vi "Compute Calibrated Phasor Array.vi"(6 "Phasor Calibration Data":T7, 7 "Phasor Calculation":T1, 8 "Error In":errorcluster, 9 "Gates Definitions":T4={"First Gate: t1"=0.0, "Gate Width: W"=0.0, "Gate Step: d"=0.0, "# Gates: G"=0.0, "Use Gate Center"=FALSE, "Frames/Image: F"=50, "Gates/Frame: L"=0, "Bits/Frame: q"=0, "Multiplicity: p"=0, "Gate Type"=enum."Square", "Gate Edge s"=4.0, "Gate Top Slope"=4.0, "Reversed Sawtooth?"=FALSE, "Computation"=FALSE, "User-defined Gate"={"X Array"=[], "Y Array"=[]}, "Tolerance"=50.0, "Integration"=enum."Item 0", "# Steps"=50.0, "Type of User-defined Function"=enum."Gate"}, 10 "Decay Definition":T2={"offset: t0"=0.0, "period: T"=0.0, "lifetime: tau"=0.0, "Incident Signal: I"=0.5, "Normalized Decays"=FALSE, "IRF Model"=enum."Dirac", "IRF Parameter 1"=0.0}, 11 "Lifetime Array":ext[](array[numeric])) -> (0 "Error Out":errorcluster, 1 "Calibrated s Array":ext[](array[numeric]), 2 "Calibrated g Array":ext[](array[numeric]), 3 "True Lifetime Array":ext[](array[numeric]), 4 "# Rejected Pairs":i32, 5 "CPU (s)":dbl)   [LabVIEW 2019]
uses:
  Phasor Calibration Data.ctl
  Gate Definitions.ctl
  Gate Type.ctl
  XY Plot Data.ctl
  Decay Definiton.ctl
  IRF Model.ctl
  Phasor Calculation Type.ctl
  SEPXP Globals.vi
panel:
  out "Uncalibrated Phasors":cxt[](array[numeric])
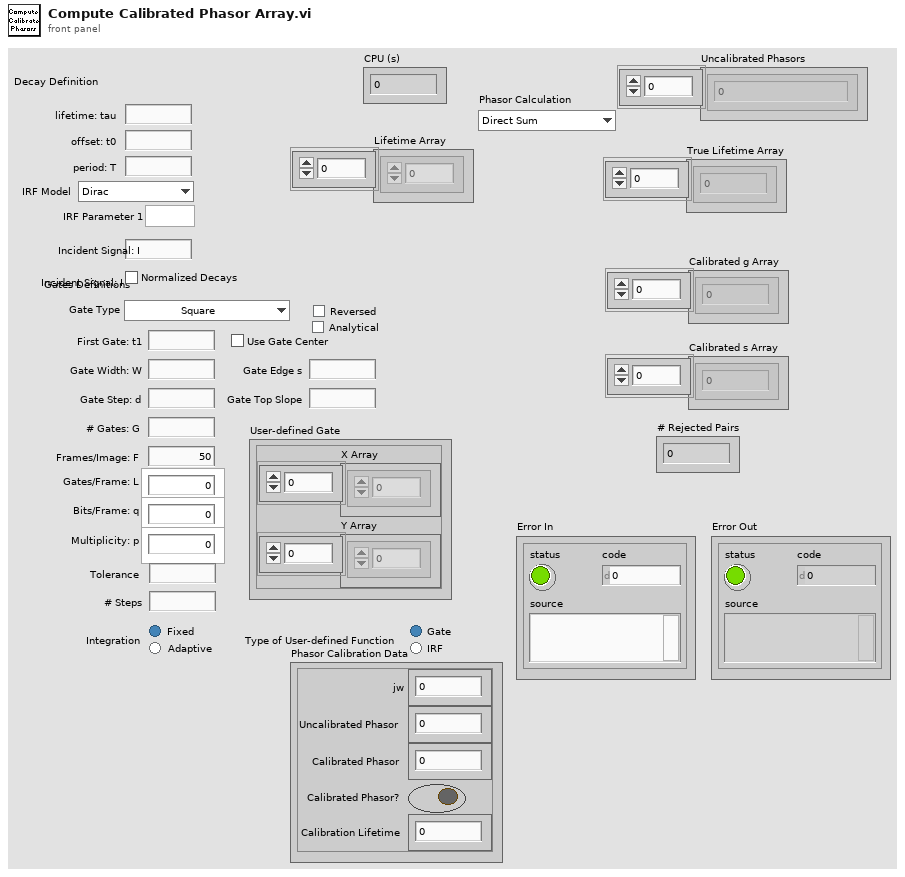
[diagram p1: front panel]
types:
  T1 = typedef "Phasor Calculation Type.ctl" = enum16{"Direct Sum", "Analytical Formula"}
  T2 = typedef "Decay Definiton.ctl" = cluster{"offset: t0":ext, "period: T":ext, "lifetime: tau":ext, "Incident Signal: I":ext, "Normalized Decays":bool, "IRF Model":T3, "IRF Parameter 1":ext}
  T3 = typedef "IRF Model.ctl" = enum16{"Dirac", "Exponential"}
  T4 = typedef "Gate Definitions.ctl" = cluster{"First Gate: t1":ext, "Gate Width: W":ext, "Gate Step: d":ext, "# Gates: G":ext, "Use Gate Center":bool, "Frames/Image: F":i32, "Gates/Frame: L":i32, "Bits/Frame: q":i32, "Multiplicity: p":i32, "Gate Type":T5, "Gate Edge s":ext, "Gate Top Slope":ext, "Reversed Sawtooth?":bool, "Computation":bool, "User-defined Gate":T6, "Tolerance":ext, "Integration":enum32{"Item 0", "Item 1"}, "# Steps":ext, "Type of User-defined Function":enum32{"Gate", "IRF"}}
  T5 = typedef "Gate Type.ctl" = enum16{"Square", "Finite Edge Square", "Finite Edge, Tilted Top Square", "Triangle", "Sawtooth", "User-defined"}
  T6 = typedef "XY Plot Data.ctl" = cluster{"X Array":dbl[], "Y Array":dbl[]}
  T7 = typedef "Phasor Calibration Data.ctl" = cluster{"jw":cxt, "Uncalibrated Phasor":cxt, "Calibrated Phasor":cxt, "Calibrated Phasor?":bool, "Calibration Lifetime":ext}
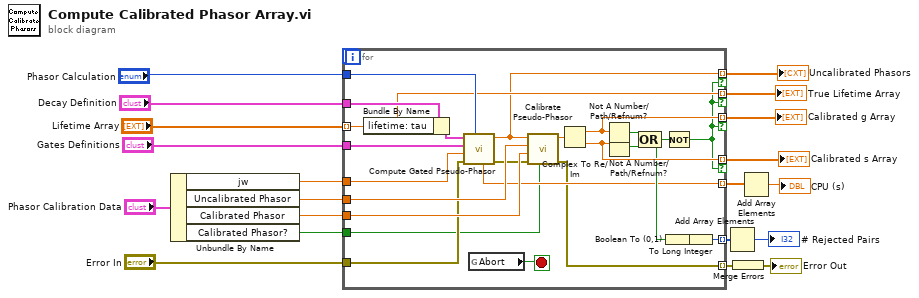
[diagram p0: block diagram]
diagram:
  n1 = Unbundle By Name("Phasor Calibration Data") -> ("jw"=w17:cxt, "Uncalibrated Phasor"=w18:cxt, "Calibrated Phasor"=w19:cxt, "Calibrated Phasor?"=w20:bool)
  n2 = for {
    tunnel: "Lifetime Array" -> [w31] mode=indexing
    tunnel: w17 -> [w43]
    tunnel: [w35] -> w11 mode=indexing if=w29
    tunnel: [w34] -> w12 mode=indexing if=w29
    tunnel: "Gates Definitions" -> [w42]
    tunnel: "Decay Definition" -> [w41]
    tunnel: w18 -> [w39]
    tunnel: w19 -> [w38]
    tunnel: w20 -> [w24]
    tunnel: "Phasor Calculation" -> [w37]
    tunnel: [w31] -> w7 mode=indexing if=w29
    tunnel: [w30] -> w6 mode=indexing if=w29
    tunnel: "Error In" -> [w36]
    tunnel: [w22] -> w8 mode=indexing
    tunnel: [w26] -> w4 mode=indexing
    tunnel: [w25] -> w2 mode=indexing
    stop <- w21 stop-if-true
    n3 = Bundle By Name(cluster=w41, "lifetime: tau"=w31) -> (w44:T2)
    n4 = call "Compute Gated Pseudo-Phasor.vi"("Phasor Calculation Type"=w37, "Error In"=w36, "j 2 pi f"=w43, "Gates Definitions"=w42, "Decay Definition"=w44) -> ("Error Out"=w23:errorcluster, "phasor"=w30:cxt, "CPU (s)"=w25:dbl)  [unwired: 4 in]
    n5 = global read "SEPXP Globals.vi" "Abort"() -> (w21:bool)
    n6 = call "Calibrate Pseudo-Phasor.vi"("Calibrated Phasor"=w24, "Error In"=w23, "Target Phasor"=w38, "Calibration Pseudo-Phasor"=w39, "Pseudo-Phasor in"=w30) -> ("Error Out"=w22:errorcluster, "Pseudo-Phasor out"=w40:cxt)  [unwired: 5 in]
    n7 = Complex To Re/Im(x + iy=w40) -> (x=w35:ext, y=w34:ext)
    n8 = Not A Number/Path/Refnum?(number/path/refnum=w35) -> (NaN/Path/Refnum?=w33:bool)
    n9 = Not A Number/Path/Refnum?(number/path/refnum=w34) -> (NaN/Path/Refnum?=w32:bool)
    n10 = Compound Arithmetic op=OR(w33, w32) -> (w28:bool)
    n11 = Boolean To (0,1)(Boolean=w28) -> (0, 1=w27:i16)
    n12 = Not(x=w28) -> (.not. x?=w29:bool)
    n13 = To Long Integer(number=w27) -> (32bit integer=w26:i32)
  }
  "Calibrated s Array" <- w12
  "Calibrated g Array" <- w11
  "True Lifetime Array" <- w7
  "Uncalibrated Phasors" <- w6
  n14 = Add Array Elements(numeric array=w4) -> (sum=→"# Rejected Pairs":i32)
  n15 = Merge Errors(w8) -> (→"Error Out":errorcluster)
  n16 = Add Array Elements(numeric array=w2) -> (sum=→"CPU (s)":dbl)
